vi "Read Config.vi"(8 "error in (no error)":errorcluster, 11 "SensorInfo in":refnum<class "SensorInfo.lvclass">) -> (0 "error out":errorcluster, 2 "Sensor Definition.lvlib:SensorConfig.lvclass":refnum<class "SensorConfig.lvclass">, 3 "SensorInfo out":refnum<class "SensorInfo.lvclass">)   [LabVIEW 2012, in "Sensor Definition.lvlib" / "SensorInfo.lvclass"]
uses:
  SensorInfo.lvclass
  SensorConfig.lvclass
  SensorInfo.lvclass/SensorInfo.ctl
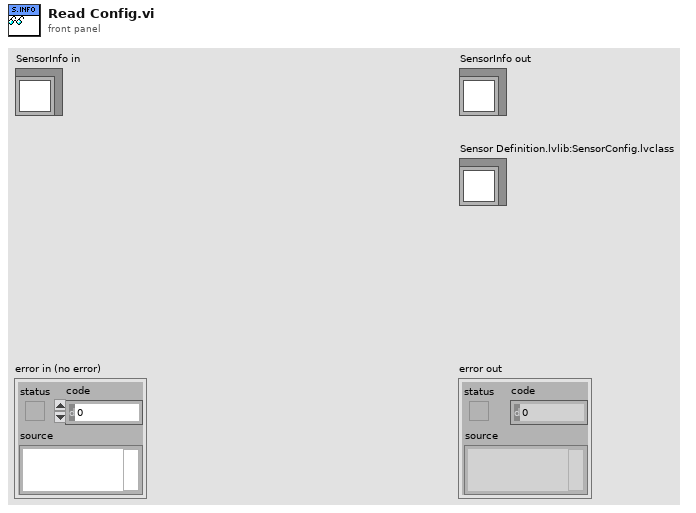
[diagram p1: front panel]
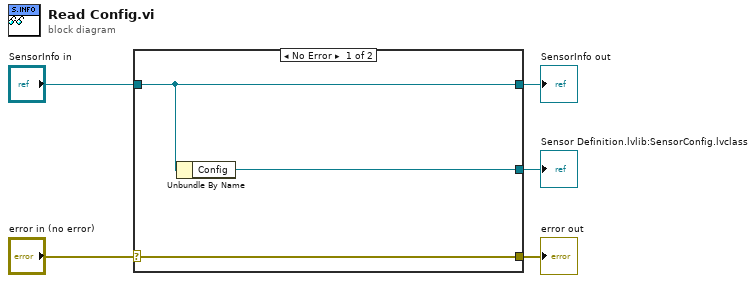
[diagram p0: block diagram]
diagram:
  n1 = case shown="No Error" "error in (no error)" {
    selector: "error in (no error)" -> [w8 w9]
    tunnel: [w8 w9] -> w4
    tunnel: [w7 w10] -> w2
    tunnel: "SensorInfo in" -> [w7 w10]
    tunnel: [w6 _] -> w1
    frame No Error {
      n2 = Unbundle By Name(w7) -> ("Config"=w6:refnum<class "SensorConfig.lvclass">)
    }
    frame Error {
    }
  }
  "error out" <- w4
  "SensorInfo out" <- w2
  "Sensor Definition.lvlib:SensorConfig.lvclass" <- w1
